vi "Periodic Tasks.vi"(8 "error in":errorcluster) -> ()   [LabVIEW 2019]
doc: "This VI runs in parallel to other tasks. It can contain as many user-defined periodic loops as you need. These can carry out PID or other sorts of timed response."
uses:
  <vilib>/Rock Robotics/WPI/Utilities/WPI_GetSetVariantRefNum.vi
  Robot Global Data.vi
  <vilib>/Rock Robotics/Network Tables/NT Read Number.vi
panel:
  out "Compressor Running":bool
  out "Compressor Monitoring":bool
  out "Motor RPM":dbl
  out "output cluster":T1
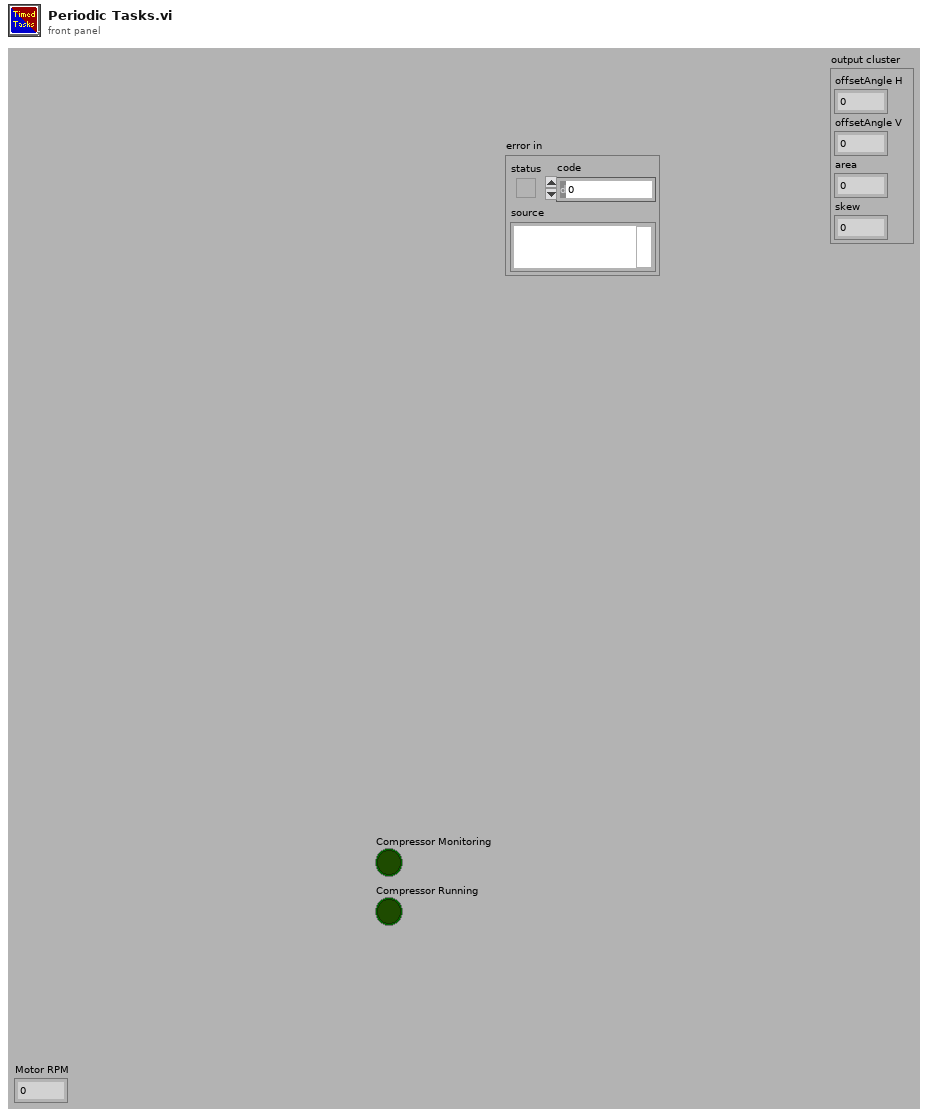
[diagram p1: front panel]
types:
  T1 = cluster{"offsetAngle H":dbl, "offsetAngle V":dbl, "area":dbl, "skew":dbl}
  T2 = typedef "WPI_JoystickDevRef.ctl" = cluster{"Device":T3}
  T3 = typedef "WPI_JoystickDeviceEnum.ctl" = enum16{"USB 0", "USB 1", "USB 2", "USB 3", "USB 4", "USB 5"}
  T4 = typedef "WPI_RobotDriveDevRef.ctl" = cluster{"DevStatus":errorcluster, "Motors[]":T5[], "Square Inputs":bool, "Max Output":dbl}
  T5 = typedef "WPI_MotorControlDeviceRef.ctl" = cluster{"DeviceStatus":errorcluster, "Type":T6, "PWM":cluster{"PWM Channel":T7, "DeadBand":T8}, "CAN":cluster{"Device Number":u8, "SetOutput VI Ref":variant, "GetOutput VI Ref":variant, "Enable VI Ref":variant, "Disable VI Ref":variant, "Data":variant}, "Invert":bool, "DIO PWM":cluster{"PWM \"Enable\" Channel":T7, "DIOChannel":T9, "PWM Rate":dbl}}
  T6 = typedef "WPI_MotorControlType.ctl" = enum16{"PWM", "CAN", "DIO PWM"}
  T7 = typedef "FPGA_DIOPWMChannel.ctl" = enum8{"PWM 0", "PWM 1", "PWM 2", "PWM 3", "PWM 4", "PWM 5", "PWM 6", "PWM 7", "PWM 8", "PWM 9", "PWM MXP 0", "PWM MXP 1", "PWM MXP 2", "PWM MXP 3", "PWM MXP 4", "PWM MXP 5", "PWM MXP 6", "PWM MXP 7", "PWM MXP 8", "PWM MXP 9", "Invalid"}
  T8 = typedef "WPI_PWMDeadband.ctl" = cluster{"Name":string, "maxPositivePwm":i32, "minPositivePwm":i32, "centerPwm":i32, "maxNegativePwm":i32, "minNegativePwm":i32, "angularRange":u16}
  T9 = typedef "FPGA_DIOChannel.ctl" = enum8{"DIO 0", "DIO 1", "DIO 2", "DIO 3", "DIO 4", "DIO 5", "DIO 6", "DIO 7", "DIO 8", "DIO 9", "DIO MXP 0", "DIO MXP 1", "DIO MXP 2", "DIO MXP 3", "DIO MXP 4", "DIO MXP 5", "DIO MXP 6", "DIO MXP 7", "DIO MXP 8", "DIO MXP 9", "DIO MXP 10", "DIO MXP 11", "DIO MXP 12", "DIO MXP 13", "DIO MXP 14", "DIO MXP 15", "SPI Port CS1", "SPI Port CS2", "SPI Port CS3", "SPI Port MISO", "SPI Port MOSI", "Invalid"}
  T10 = typedef "WPI_CompressorDevRef.ctl" = cluster{"DevStatus":errorcluster, "Pneumatics Control Module":u8}
  T11 = cluster{"JoystickDevRef":T2, "RobotDriveDevRef":T4, "MotorControlDevRef":T5, "CompressorDevRef":T10}
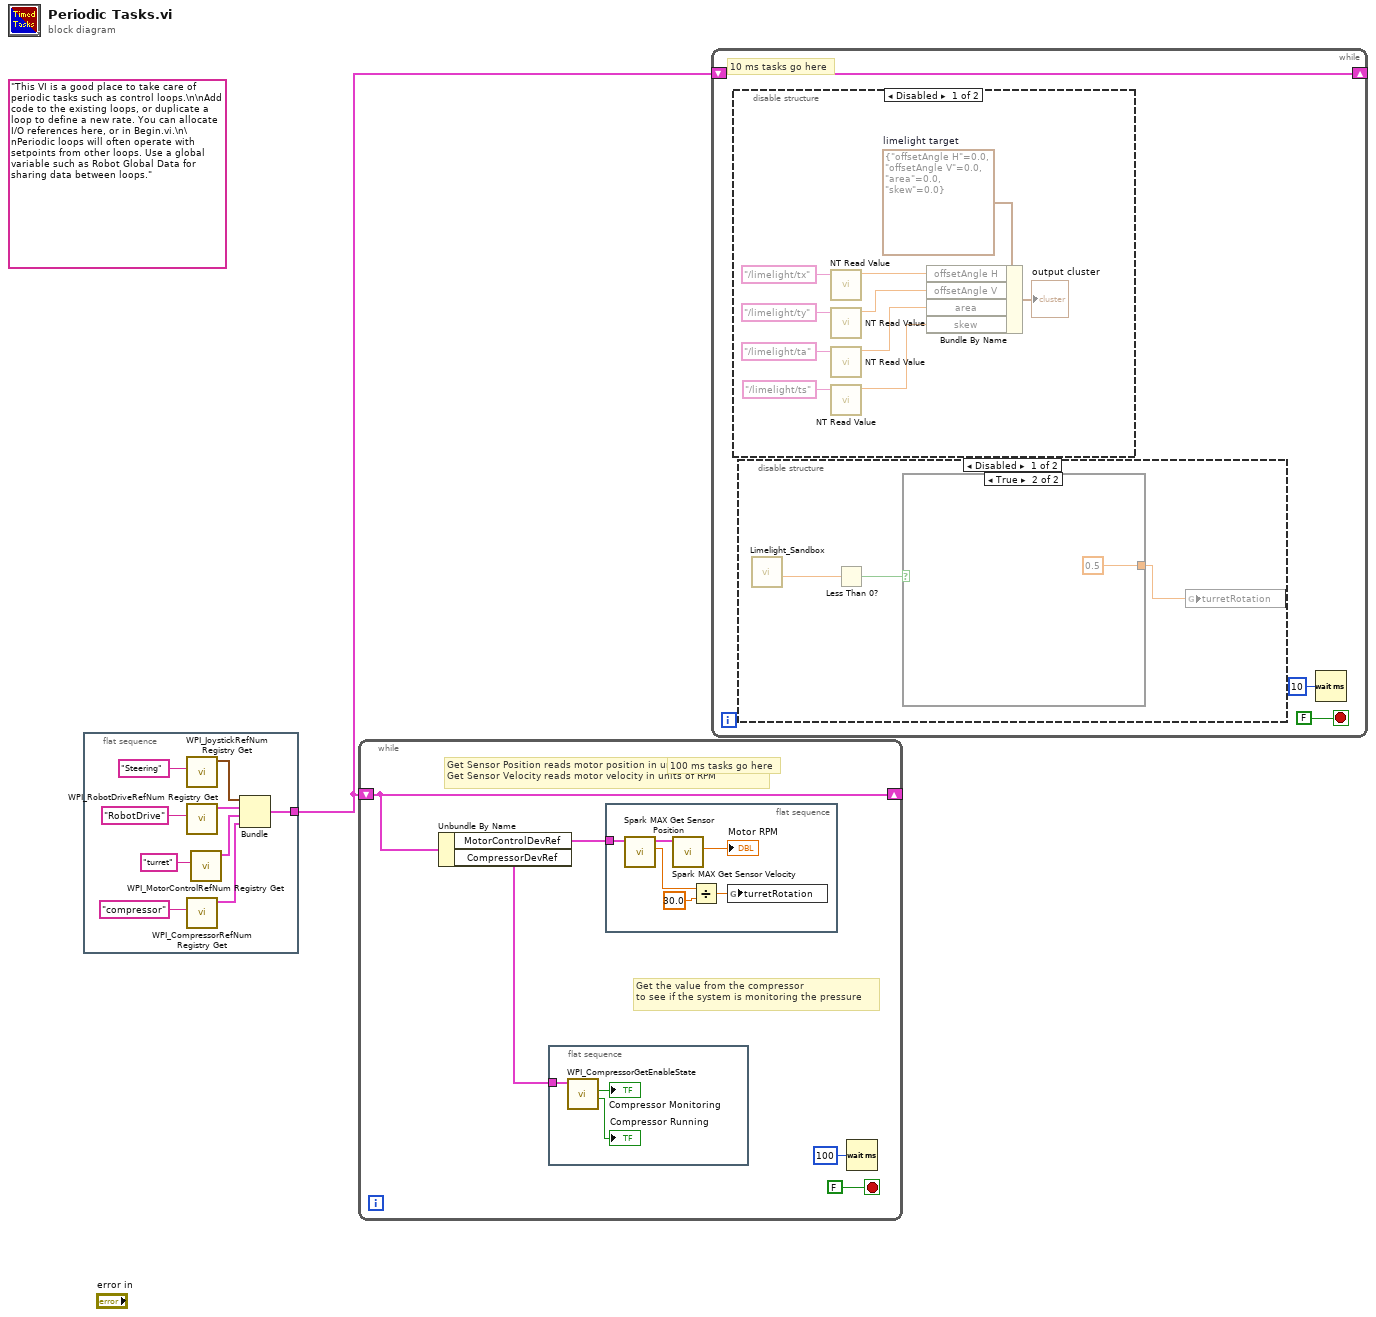
[diagram p0: block diagram]
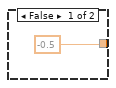
[diagram p2: hidden frame]
diagram:
  (unwired) "This VI is a good place to take care of periodic tasks such as control loops.\n\nAdd code to the existing loops, or duplicate a loop to define a new rate. You can allocate I/O references here, or in Begin.vi.\n\nPeriodic loops will often operate with setpoints from other loops. Use a global variable such as Robot Global Data for sharing data between loops."
  n1 = flat-sequence {
    tunnel: [w6] -> w1
    frame #0 {
      n2 = call <vilib>:"WPI_JoystickRefNum Registry Get.vi"("refnum name"="Steering") -> ("JoystickDevRef"=w8:T2)  [unwired: 1 in, 9 out]
      n3 = call <vilib>:"WPI_RobotDriveRefNum Registry Get.vi"("refnum name"="RobotDrive") -> ("RobotDriveDevRef"=w7:T4)  [unwired: 1 in, 9 out]
      n4 = call <vilib>:"WPI_CompressorRefNum Registry Get.vi"("refnum name"="compressor") -> ("CompressorDevRef"=w2:T10)  [unwired: 9 in, 1 out]
      n5 = call <vilib>:"WPI_MotorControlRefNum Registry Get.vi"("refnum name"="turret") -> ("MotorControlDevRef"=w4:T5)  [unwired: 9 in, 1 out]
      n6 = Bundle("JoystickDevRef"=w8, "RobotDriveDevRef"=w7, "MotorControlDevRef"=w4, "CompressorDevRef"=w2) -> (w6:T11)  [unwired: 1 out]
    }
  }
  n7 = while {
    shift-right: [w12] -> _
    shift-left: w1 -> [w12]
    stop <- FALSE stop-if-true
    # "Get the value from the compressor \nto see if the system is monitoring the pressure"
    # "Get Sensor Position reads motor position in units of rotations\nGet Sensor Velocity reads motor velocity in units of RPM"
    # "100 ms tasks go here"
    n8 = Unbundle By Name(w12) -> ("MotorControlDevRef"=w13:T5, "CompressorDevRef"=w11:T10)
    n9 = flat-sequence {
      tunnel: w11 -> [w16]
      frame #0 {
        n10 = call <vilib>:"WPI_CompressorGetEnableState.vi"("CompressorDevRef"=w16) -> ("Compressor Running"=→"Compressor Running":bool, "Enabled"=→"Compressor Monitoring":bool)  [unwired: 1 in, 8 out]
      }
    }
    n11 = flat-sequence {
      tunnel: w13 -> [w24]
      frame #0 {
        n12 = call <vilib>:"Spark MAX Get Sensor Position.vi"("MotorControlDevRef in"=w24) -> ("Sensor Position"=w21:dbl, "MotorControlDevRef out"=w23:T5)  [unwired: 7 in, 2 out]
        n13 = call <vilib>:"Spark MAX Get Sensor Velocity.vi"("MotorControlDevRef in"=w23) -> ("Sensor Velocity"=→"Motor RPM":dbl)  [unwired: 7 in, 3 out]
        n14 = Divide(x=w21, y=30.0) -> (x/y=w19:dbl)
        n15 = global write "Robot Global Data.vi" "turretRotation"(w19) -> ()
      }
    }
    n16 = Wait (ms)(milliseconds to wait=u32 100) -> ()  [unwired: 1 out]
  }
  n17 = while {
    shift-right: [w25] -> _
    shift-left: w1 -> [w25]
    stop <- FALSE stop-if-true
    # "10 ms tasks go here"
    n18 = disable-structure shown="Disabled" {
      frame Disabled {
        w38 = T1 {"offsetAngle H"=0.0, "offsetAngle V"=0.0, "area"=0.0, "skew"=0.0}  # limelight target
        n19 = call-poly <vilib>:"NT Read Value.vi"("Name"="/limelight/tx") -> ("Numeric"=w37:dbl)  [unwired: 9 in, 1 out]
        n20 = call-poly <vilib>:"NT Read Value.vi"("Name"="/limelight/ty") -> ("Numeric"=w36:dbl)  [unwired: 9 in, 1 out]
        n21 = call-poly <vilib>:"NT Read Value.vi"("Name"="/limelight/ta") -> ("Numeric"=w35:dbl)  [unwired: 9 in, 1 out]
        n22 = call-poly <vilib>:"NT Read Value.vi"("Name"="/limelight/ts") -> ("Numeric"=w34:dbl)  [unwired: 9 in, 1 out]
        n23 = Bundle By Name(cluster=w38, "offsetAngle H"=w37, "offsetAngle V"=w36, "area"=w35, "skew"=w34) -> (→"output cluster":T1)
      }
      frame Enabled {
      }
    }
    n24 = disable-structure shown="Disabled" {
      frame Disabled {
        n25 = call "Limelight_Sandbox.vi"() -> ("limelightTX"=w30:dbl)  [unwired: 9 in, 2 out]
        n26 = Less Than 0?(x=w30) -> (x < 0?=w29:bool)
        n27 = case shown="True" w29 {
          tunnel: [-0.5 ("Output") 0.5 ("Output")] -> w28
          frame False {
          }
          frame True {
          }
        }
        n28 = global write "Robot Global Data.vi" "turretRotation"(w28) -> ()
      }
      frame Enabled {
      }
    }
    n29 = Wait (ms)(milliseconds to wait=u32 10) -> ()  [unwired: 1 out]
  }
